vi "电流方向控制-PLC - 副本.vi"() -> ()   [LabVIEW 2021]
panel:
  in  "停止":bool
  in  "?":T1
  in  "PLC地址":string="192.168.100.10"
  out "?":bool
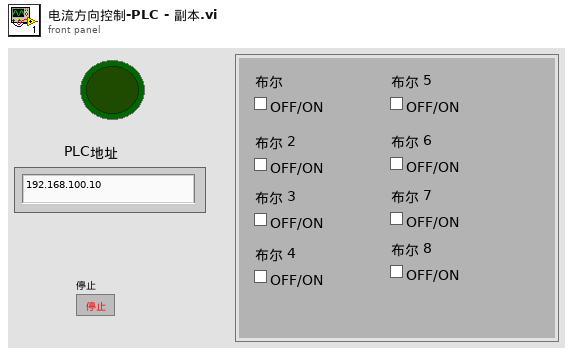
[diagram p1: front panel]
types:
  T1 = cluster{"布尔":bool, "布尔 2":bool, "布尔 3":bool, "布尔 4":bool, "布尔 5":bool, "布尔 6":bool, "布尔 7":bool, "布尔 8":bool}
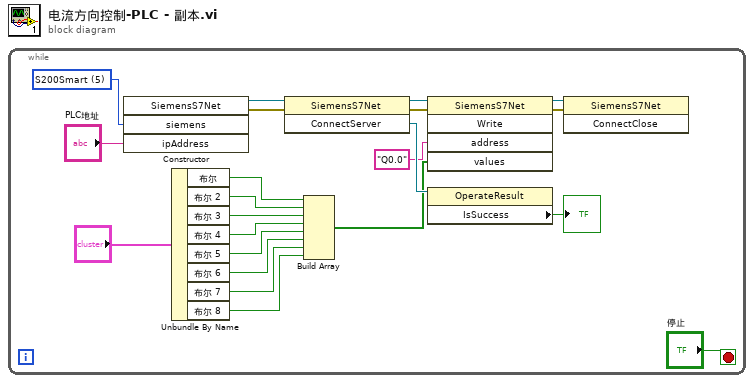
[diagram p0: block diagram]
diagram:
  n1 = while {
    stop <- "停止" stop-if-true
    w12 = 5 items=["S1200"=1, "S300"=2, "S400"=3, "S1500"=4, "S200Smart"=5, "S200"=6] ("siemens")
    n2 = constructor class="SiemensS7Net"("siemens"=w12, "ipAddress"="PLC地址") -> (reference out=w21:refnum<k24>, error out=w22:errorcluster)  [unwired: 3 in, 3 out]
    n3 = Unbundle By Name("?") -> ("布尔"=w9:bool, "布尔 2"=w8:bool, "布尔 3"=w7:bool, "布尔 4"=w6:bool, "布尔 5"=w5:bool, "布尔 6"=w4:bool, "布尔 7"=w3:bool, "布尔 8"=w2:bool)
    n4 = invoke class="SiemensS7Net" method="ConnectServer"(reference=w21, error in=w22) -> (reference out=w17:refnum<k24>, error out=w16:errorcluster, "ConnectServer"=w19:refnum<k24>)  [unwired: 1 in]
    n5 = Build Array(w9, w8, w7, w6, w5, w4, w3, w2) -> (w13:bool[])
    n6 = invoke class="SiemensS7Net" method="Write"(reference=w17, error in=w16, "address"="Q0.0", "values"=w13) -> (reference out=w14:refnum<k24>, error out=w15:errorcluster)  [unwired: 1 in, 3 out]
    n7 = property class="OperateResult"(reference=w19) -> ("IsSuccess"=→"?":bool)  [unwired: 1 in, 2 out]
    n8 = invoke class="SiemensS7Net" method="ConnectClose"(reference=w14, error in=w15) -> ()  [unwired: 1 in, 3 out]
  }
